vi "50 Modify 1 to -1 Input.vi"() -> ()   [LabVIEW 2018]
panel:
  in  "stop":bool
  in  "Method":i32
  out "Output":dbl(slide) scale=0.0..1.0
  in  "Joystick":dbl(slide) scale=1.0..-1.0
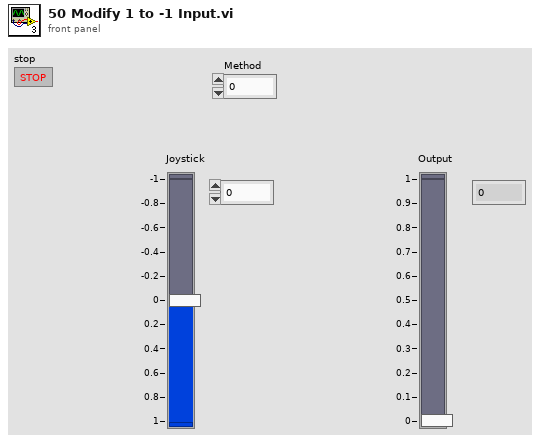
[diagram p1: front panel]
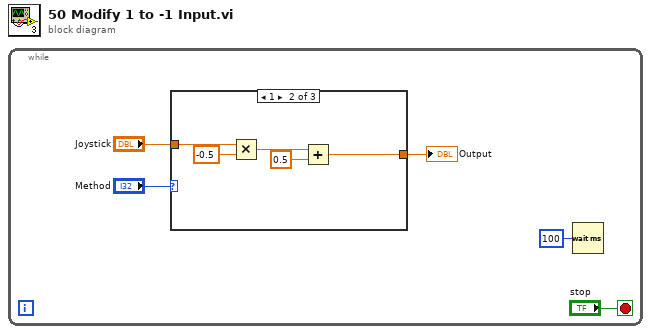
[diagram p0: block diagram]
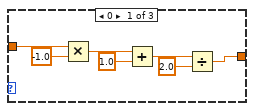
[diagram p2: hidden frame]
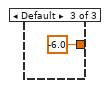
[diagram p3: hidden frame]
diagram:
  n1 = while {
    stop <- "stop" stop-if-true
    n2 = case shown="1" "Method" {
      tunnel: "Joystick" -> [w12 w17 _]
      tunnel: [w6 w13 -6.0] -> w4
      frame 0 {
        n3 = Multiply(x=w12, y=-1.0) -> (x*y=w10:dbl)
        n4 = Add(x=w10, y=1.0) -> (x+y=w8:dbl)
        n5 = Divide(x=w8, y=2.0) -> (x/y=w6:dbl)
      }
      frame 1 {
        n6 = Multiply(x=w17, y=-0.5) -> (x*y=w15:dbl)
        n7 = Add(x=w15, y=0.5) -> (x+y=w13:dbl)
      }
      frame Default {
      }
    }
    "Output" <- w4
    n8 = Wait (ms)(milliseconds to wait=u32 100) -> ()  [unwired: 1 out]
  }
